vi "App - analyze RUS V6.vi"() -> ()   [LabVIEW 2015] (continued)
"mod time(min)"=58229664.733333334, "file format"=enum."binary", "power(V)"=2.1, "Magn Field(T) "=0.0}, {"temperature"=77.2, "temperature str"="77.20000", "file path"=path "D:/Data/Ultrasound/LSCO/LSCO22__130814c/5_Cooling_2nd_try/September_2014/091714/77.20000K_500_2500_2.10000V_0.00000T_Sep17-2014__02-26-03_001_091714.bin", "last mod"=timestamp(3493779963 s since 1904-01-01), "file name str"="D:\\Data\\Ultrasound\\LSCO\\LSCO22__130814c\\5_Cooling_2nd_try\\September_2014\\091714\\77.20000K_500_2500_2.10000V_0.00000T_Sep17-2014__02-26-03_001_091714.bin", "mod time(min)"=58229666.05, "file format"=enum."binary", "power(V)"=2.1, "Magn Field(T) "=0.0}, {"temperature"=77.118, "temperature str"="77.11800", "file path"=path "D:/Data/Ultrasound/LSCO/LSCO22__130814c/5_Cooling_2nd_try/September_2014/091714/77.11800K_500_2500_2.10000V_0.00000T_Sep17-2014__02-27-22_001_091714.bin", "last mod"=timestamp(3493780042 s since 1904-01-01), "file name str"="D:\\Data\\Ultrasound\\LSCO\\LSCO22__130814c\\5_Cooling_2nd_try\\September_2014\\091714\\77.11800K_500_2500_2.10000V_0.00000T_Sep17-2014__02-27-22_001_091714.bin", "mod time(min)"=58229667.36666667, "file format"=enum."binary", "power(V)"=2.1, "Magn Field(T) "=0.0}, {"temperature"=77.043, "temperature str"="77.04300", "file path"=path "D:/Data/Ultrasound/LSCO/LSCO22__130814c/5_Cooling_2nd_try/September_2014/091714/77.04300K_500_2500_2.10000V_0.00000T_Sep17-2014__02-28-42_001_091714.bin", "last mod"=timestamp(3493780122 s since 1904-01-01), "file name str"="D:\\Data\\Ultrasound\\LSCO\\LSCO22__130814c\\5_Cooling_2nd_try\\September_2014\\091714\\77.04300K_500_2500_2.10000V_0.00000T_Sep17-2014__02-28-42_001_091714.bin", "mod time(min)"=58229668.7, "file format"=enum."binary", "power(V)"=2.1, "Magn Field(T) "=0.0}, {"temperature"=76.965, "temperature str"="76.96500", "file path"=path "D:/Data/Ultrasound/LSCO/LSCO22__130814c/5_Cooling_2nd_try/September_2014/091714/76.96500K_500_2500_2.10000V_0.00000T_Sep17-2014__02-30-01_001_091714.bin", "last mod"=timestamp(3493780201 s since 1904-01-01), "file name str"="D:\\Data\\Ultrasound\\LSCO\\LSCO22__130814c\\5_Cooling_2nd_try\\September_2014\\091714\\76.96500K_500_2500_2.10000V_0.00000T_Sep17-2014__02-30-01_001_091714.bin", "mod time(min)"=58229670.016666666, "file format"=enum."binary", "power(V)"=2.1, "Magn Field(T) "=0.0}, {"temperature"=76.89, "temperature str"="76.89000", "file path"=path "D:/Data/Ultrasound/LSCO/LSCO22__130814c/5_Cooling_2nd_try/September_2014/091714/76.89000K_500_2500_2.10000V_0.00000T_Sep17-2014__02-31-21_001_091714.bin", "last mod"=timestamp(3493780281 s since 1904-01-01), "file name str"="D:\\Data\\Ultrasound\\LSCO\\LSCO22__130814c\\5_Cooling_2nd_try\\September_2014\\091714\\76.89000K_500_2500_2.10000V_0.00000T_Sep17-2014__02-31-21_001_091714.bin", "mod time(min)"=58229671.35, "file format"=enum."binary", "power(V)"=2.1, "Magn Field(T) "=0.0}, {"temperature"=76.811, "temperature str"="76.81100", "file path"=path "D:/Data/Ultrasound/LSCO/LSCO22__130814c/5_Cooling_2nd_try/September_2014/091714/76.81100K_500_2500_2.10000V_0.00000T_Sep17-2014__02-32-40_001_091714.bin", "last mod"=timestamp(3493780360 s since 1904-01-01), "file name str"="D:\\Data\\Ultrasound\\LSCO\\LSCO22__130814c\\5_Cooling_2nd_try\\September_2014\\091714\\76.81100K_500_2500_2.10000V_0.00000T_Sep17-2014__02-32-40_001_091714.bin", "mod time(min)"=58229672.666666664, "file format"=enum."binary", "power(V)"=2.1, "Magn Field(T) "=0.0}, {"temperature"=76.733, "temperature str"="76.73300", "file path"=path "D:/Data/Ultrasound/LSCO/LSCO22__130814c/5_Cooling_2nd_try/September_2014/091714/76.73300K_500_2500_2.10000V_0.00000T_Sep17-2014__02-33-59_001_091714.bin", "last mod"=timestamp(3493780439 s since 1904-01-01), "file name str"="D:\\Data\\Ultrasound\\LSCO\\LSCO22__130814c\\5_Cooling_2nd_try\\September_2014\\091714\\76.73300K_500_2500_2.10000V_0.00000T_Sep17-2014__02-33-59_001_091714.bin", "mod time(min)"=58229673.983333334, "file format"=enum."binary", "power(V)"=2.1, "Magn Field(T) "=0.0}, {"temperature"=76.659, "temperature str"="76.65900", "file path"=path "D:/Data/Ultrasound/LSCO/LSCO22__130814c/5_Cooling_2nd_try/September_2014/091714/76.65900K_500_2500_2.10000V_0.00000T_Sep17-2014__02-35-19_001_091714.bin", "last mod"=timestamp(3493780519 s since 1904-01-01), "file name str"="D:\\Data\\Ultrasound\\LSCO\\LSCO22__130814c\\5_Cooling_2nd_try\\September_2014\\091714\\76.65900K_500_2500_2.10000V_0.00000T_Sep17-2014__02-35-19_001_091714.bin", "mod time(min)"=58229675.31666667, "file format"=enum."binary", "power(V)"=2.1, "Magn Field(T) "=0.0}, {"temperature"=76.581, "temperature str"="76.58100", "file path"=path "D:/Data/Ultrasound/LSCO/LSCO22__130814c/5_Cooling_2nd_try/September_2014/091714/76.58100K_500_2500_2.10000V_0.00000T_Sep17-2014__02-36-38_001_091714.bin", "last mod"=timestamp(3493780598 s since 1904-01-01), "file name str"="D:\\Data\\Ultrasound\\LSCO\\LSCO22__130814c\\5_Cooling_2nd_try\\September_2014\\091714\\76.58100K_500_2500_2.10000V_0.00000T_Sep17-2014__02-36-38_001_091714.bin", "mod time(min)"=58229676.63333333, "file format"=enum."binary", "power(V)"=2.1, "Magn Field(T) "=0.0}, {"temperature"=76.505, "temperature str"="76.50500", "file path"=path "D:/Data/Ultrasound/LSCO/LSCO22__130814c/5_Cooling_2nd_try/September_2014/091714/76.50500K_500_2500_2.10000V_0.00000T_Sep17-2014__02-37-58_001_091714.bin", "last mod"=timestamp(3493780678 s since 1904-01-01), "file name str"="D:\\Data\\Ultrasound\\LSCO\\LSCO22__130814c\\5_Cooling_2nd_try\\September_2014\\091714\\76.50500K_500_2500_2.10000V_0.00000T_Sep17-2014__02-37-58_001_091714.bin", "mod time(min)"=58229677.96666667, "file format"=enum."binary", "power(V)"=2.1, "Magn Field(T) "=0.0}, {"temperature"=76.428, "temperature str"="76.42800", "file path"=path "D:/Data/Ultrasound/LSCO/LSCO22__130814c/5_Cooling_2nd_try/September_2014/091714/76.42800K_500_2500_2.10000V_0.00000T_Sep17-2014__02-39-17_001_091714.bin", "last mod"=timestamp(3493780757 s since 1904-01-01), "file name str"="D:\\Data\\Ultrasound\\LSCO\\LSCO22__130814c\\5_Cooling_2nd_try\\September_2014\\091714\\76.42800K_500_2500_2.10000V_0.00000T_Sep17-2014__02-39-17_001_091714.bin", "mod time(min)"=58229679.28333333, "file format"=enum."binary", "power(V)"=2.1, "Magn Field(T) "=0.0}, {"temperature"=76.351, "temperature str"="76.35100", "file path"=path "D:/Data/Ultrasound/LSCO/LSCO22__130814c/5_Cooling_2nd_try/September_2014/091714/76.35100K_500_2500_2.10000V_0.00000T_Sep17-2014__02-40-36_001_091714.bin", "last mod"=timestamp(3493780836 s since 1904-01-01), "file name str"="D:\\Data\\Ultrasound\\LSCO\\LSCO22__130814c\\5_Cooling_2nd_try\\September_2014\\091714\\76.35100K_500_2500_2.10000V_0.00000T_Sep17-2014__02-40-36_001_091714.bin", "mod time(min)"=58229680.6, "file format"=enum."binary", "power(V)"=2.1, "Magn Field(T) "=0.0}, {"temperature"=76.277, "temperature str"="76.27700", "file path"=path "D:/Data/Ultrasound/LSCO/LSCO22__130814c/5_Cooling_2nd_try/September_2014/091714/76.27700K_500_2500_2.10000V_0.00000T_Sep17-2014__02-41-56_001_091714.bin", "last mod"=timestamp(3493780916 s since 1904-01-01), "file name str"="D:\\Data\\Ultrasound\\LSCO\\LSCO22__130814c\\5_Cooling_2nd_try\\September_2014\\091714\\76.27700K_500_2500_2.10000V_0.00000T_Sep17-2014__02-41-56_001_091714.bin", "mod time(min)"=58229681.93333333, "file format"=enum."binary", "power(V)"=2.1, "Magn Field(T) "=0.0}, {"temperature"=76.2, "temperature str"="76.20000", "file path"=path "D:/Data/Ultrasound/LSCO/LSCO22__130814c/5_Cooling_2nd_try/September_2014/091714/76.20000K_500_2500_2.10000V_0.00000T_Sep17-2014__02-43-15_001_091714.bin", "last mod"=timestamp(3493780995 s since 1904-01-01), "file name str"="D:\\Data\\Ultrasound\\LSCO\\LSCO22__130814c\\5_Cooling_2nd_try\\September_2014\\091714\\76.20000K_500_2500_2.10000V_0.00000T_Sep17-2014__02-43-15_001_091714.bin", "mod time(min)"=58229683.25, "file format"=enum."binary", "power(V)"=2.1, "Magn Field(T) "=0.0}, {"temperature"=76.124, "temperature str"="76.12400", "file path"=path "D:/Data/Ultrasound/LSCO/LSCO22__130814c/5_Cooling_2nd_try/September_2014/091714/76.12400K_500_2500_2.10000V_0.00000T_Sep17-2014__02-44-34_001_091714.bin", "last mod"=timestamp(3493781074 s since 1904-01-01), "file name str"="D:\\Data\\Ultrasound\\LSCO\\LSCO22__130814c\\5_Cooling_2nd_try\\September_2014\\091714\\76.12400K_500_2500_2.10000V_0.00000T_Sep17-2014__02-44-34_001_091714.bin", "mod time(min)"=58229684.56666667, "file format"=enum."binary", "power(V)"=2.1, "Magn Field(T) "=0.0}, {"temperature"=76.051, "temperature str"="76.05100", "file path"=path "D:/Data/Ultrasound/LSCO/LSCO22__130814c/5_Cooling_2nd_try/September_2014/091714/76.05100K_500_2500_2.10000V_0.00000T_Sep17-2014__02-45-54_001_091714.bin", "last mod"=timestamp(3493781154 s since 1904-01-01), "file name str"="D:\\Data\\Ultrasound\\LSCO\\LSCO22__130814c\\5_Cooling_2nd_try\\September_2014\\091714\\76.05100K_500_2500_2.10000V_0.00000T_Sep17-2014__02-45-54_001_091714.bin", "mod time(min)"=58229685.9, "file format"=enum."binary", "power(V)"=2.1, "Magn Field(T) "=0.0}, {"temperature"=75.976, "temperature str"="75.97600", "file path"=path "D:/Data/Ultrasound/LSCO/LSCO22__130814c/5_Cooling_2nd_try/September_2014/091714/75.97600K_500_2500_2.10000V_0.00000T_Sep17-2014__02-47-13_001_091714.bin", "last mod"=timestamp(3493781233 s since 1904-01-01), "file name str"="D:\\Data\\Ultrasound\\LSCO\\LSCO22__130814c\\5_Cooling_2nd_try\\September_2014\\091714\\75.97600K_500_2500_2.10000V_0.00000T_Sep17-2014__02-47-13_001_091714.bin", "mod time(min)"=58229687.21666667, "file format"=enum."binary", "power(V)"=2.1, "Magn Field(T) "=0.0}, {"temperature"=75.901, "temperature str"="75.90100", "file path"=path "D:/Data/Ultrasound/LSCO/LSCO22__130814c/5_Cooling_2nd_try/September_2014/091714/75.90100K_500_2500_2.10000V_0.00000T_Sep17-2014__02-48-33_001_091714.bin", "last mod"=timestamp(3493781313 s since 1904-01-01), "file name str"="D:\\Data\\Ultrasound\\LSCO\\LSCO22__130814c\\5_Cooling_2nd_try\\September_2014\\091714\\75.90100K_500_2500_2.10000V_0.00000T_Sep17-2014__02-48-33_001_091714.bin", "mod time(min)"=58229688.55, "file format"=enum."binary", "power(V)"=2.1, "Magn Field(T) "=0.0}, {"temperature"=75.826, "temperature str"="75.82600", "file path"=path "D:/Data/Ultrasound/LSCO/LSCO22__130814c/5_Cooling_2nd_try/September_2014/091714/75.82600K_500_2500_2.10000V_0.00000T_Sep17-2014__02-49-52_001_091714.bin", "last mod"=timestamp(3493781392 s since 1904-01-01), "file name str"="D:\\Data\\Ultrasound\\LSCO\\LSCO22__130814c\\5_Cooling_2nd_try\\September_2014\\091714\\75.82600K_500_2500_2.10000V_0.00000T_Sep17-2014__02-49-52_001_091714.bin", "mod time(min)"=58229689.86666667, "file format"=enum."binary", "power(V)"=2.1, "Magn Field(T) "=0.0}, {"temperature"=75.75, "temperature str"="75.75000", "file path"=path "D:/Data/Ultrasound/LSCO/LSCO22__130814c/5_Cooling_2nd_try/September_2014/091714/75.75000K_500_2500_2.10000V_0.00000T_Sep17-2014__02-51-11_001_091714.bin", "last mod"=timestamp(3493781471 s since 1904-01-01), "file name str"="D:\\Data\\Ultrasound\\LSCO\\LSCO22__130814c\\5_Cooling_2nd_try\\September_2014\\091714\\75.75000K_500_2500_2.10000V_0.00000T_Sep17-2014__02-51-11_001_091714.bin", "mod time(min)"=58229691.18333333, "file format"=enum."binary", "power(V)"=2.1, "Magn Field(T) "=0.0}, {"temperature"=75.678, "temperature str"="75.67800", "file path"=path "D:/Data/Ultrasound/LSCO/LSCO22__130814c/5_Cooling_2nd_try/September_2014/091714/75.67800K_500_2500_2.10000V_0.00000T_Sep17-2014__02-52-31_001_091714.bin", "last mod"=timestamp(3493781551 s since 1904-01-01), "file name str"="D:\\Data\\Ultrasound\\LSCO\\LSCO22__130814c\\5_Cooling_2nd_try\\September_2014\\091714\\75.67800K_500_2500_2.10000V_0.00000T_Sep17-2014__02-52-31_001_091714.bin", "mod time(min)"=58229692.516666666, "file format"=enum."binary", "power(V)"=2.1, "Magn Field(T) "=0.0}, {"temperature"=75.603, "temperature str"="75.60300", "file path"=path "D:/Data/Ultrasound/LSCO/LSCO22__130814c/5_Cooling_2nd_try/September_2014/091714/75.60300K_500_2500_2.10000V_0.00000T_Sep17-2014__02-53-50_001_091714.bin", "last mod"=timestamp(3493781630 s since 1904-01-01), "file name str"="D:\\Data\\Ultrasound\\LSCO\\LSCO22__130814c\\5_Cooling_2nd_try\\September_2014\\091714\\75.60300K_500_2500_2.10000V_0.00000T_Sep17-2014__02-53-50_001_091714.bin", "mod time(min)"=58229693.833333336, "file format"=enum."binary", "power(V)"=2.1, "Magn Field(T) "=0.0}, {"temperature"=75.531, "temperature str"="75.53100", "file path"=path "D:/Data/Ultrasound/LSCO/LSCO22__130814c/5_Cooling_2nd_try/September_2014/091714/75.53100K_500_2500_2.10000V_0.00000T_Sep17-2014__02-55-09_001_091714.bin", "last mod"=timestamp(3493781709 s since 1904-01-01), "file name str"="D:\\Data\\Ultrasound\\LSCO\\LSCO22__130814c\\5_Cooling_2nd_try\\September_2014\\091714\\75.53100K_500_2500_2.10000V_0.00000T_Sep17-2014__02-55-09_001_091714.bin", "mod time(min)"=58229695.15, "file format"=enum."binary", "power(V)"=2.1, "Magn Field(T) "=0.0}, {"temperature"=75.457, "temperature str"="75.45700", "file path"=path "D:/Data/Ultrasound/LSCO/LSCO22__130814c/5_Cooling_2nd_try/September_2014/091714/75.45700K_500_2500_2.10000V_0.00000T_Sep17-2014__02-56-29_001_091714.bin", "last mod"=timestamp(3493781789 s since 1904-01-01), "file name str"="D:\\Data\\Ultrasound\\LSCO\\LSCO22__130814c\\5_Cooling_2nd_try\\September_2014\\091714\\75.45700K_500_2500_2.10000V_0.00000T_Sep17-2014__02-56-29_001_091714.bin", "mod time(min)"=58229696.483333334, "file format"=enum."binary", "power(V)"=2.1, "Magn Field(T) "=0.0}, {"temperature"=75.379, "temperature str"="75.37900", "file path"=path "D:/Data/Ultrasound/LSCO/LSCO22__130814c/5_Cooling_2nd_try/September_2014/091714/75.37900K_500_2500_2.10000V_0.00000T_Sep17-2014__02-57-48_001_091714.bin", "last mod"=timestamp(3493781868 s since 1904-01-01), "file name str"="D:\\Data\\Ultrasound\\LSCO\\LSCO22__130814c\\5_Cooling_2nd_try\\September_2014\\091714\\75.37900K_500_2500_2.10000V_0.00000T_Sep17-2014__02-57-48_001_091714.bin", "mod time(min)"=58229697.8, "file format"=enum."binary", "power(V)"=2.1, "Magn Field(T) "=0.0}, {"temperature"=75.31, "temperature str"="75.31000", "file path"=path "D:/Data/Ultrasound/LSCO/LSCO22__130814c/5_Cooling_2nd_try/September_2014/091714/75.31000K_500_2500_2.10000V_0.00000T_Sep17-2014__02-59-08_001_091714.bin", "last mod"=timestamp(3493781948 s since 1904-01-01), "file name str"="D:\\Data\\Ultrasound\\LSCO\\LSCO22__130814c\\5_Cooling_2nd_try\\September_2014\\091714\\75.31000K_500_2500_2.10000V_0.00000T_Sep17-2014__02-59-08_001_091714.bin", "mod time(min)"=58229699.13333333, "file format"=enum."binary", "power(V)"=2.1, "Magn Field(T) "=0.0}, {"temperature"=75.236, "temperature str"="75.23600", "file path"=path "D:/Data/Ultrasound/LSCO/LSCO22__130814c/5_Cooling_2nd_try/September_2014/091714/75.23600K_500_2500_2.10000V_0.00000T_Sep17-2014__03-00-27_001_091714.bin", "last mod"=timestamp(3493782027 s since 1904-01-01), "file name str"="D:\\Data\\Ultrasound\\LSCO\\LSCO22__130814c\\5_Cooling_2nd_try\\September_2014\\091714\\75.23600K_500_2500_2.10000V_0.00000T_Sep17-2014__03-00-27_001_091714.bin", "mod time(min)"=58229700.45, "file format"=enum."binary", "power(V)"=2.1, "Magn Field(T) "=0.0}, {"temperature"=75.165, "temperature str"="75.16500", "file path"=path "D:/Data/Ultrasound/LSCO/LSCO22__130814c/5_Cooling_2nd_try/September_2014/091714/75.16500K_500_2500_2.10000V_0.00000T_Sep17-2014__03-01-46_001_091714.bin", "last mod"=timestamp(3493782106 s since 1904-01-01), "file name str"="D:\\Data\\Ultrasound\\LSCO\\LSCO22__130814c\\5_Cooling_2nd_try\\September_2014\\091714\\75.16500K_500_2500_2.10000V_0.00000T_Sep17-2014__03-01-46_001_091714.bin", "mod time(min)"=58229701.766666666, "file format"=enum."binary", "power(V)"=2.1, "Magn Field(T) "=0.0}, {"temperature"=75.09, "temperature str"="75.09000", "file path"=path "D:/Data/Ultrasound/LSCO/LSCO22__130814c/5_Cooling_2nd_try/September_2014/091714/75.09000K_500_2500_2.10000V_0.00000T_Sep17-2014__03-03-06_001_091714.bin", "last mod"=timestamp(3493782186 s since 1904-01-01), "file name str"="D:\\Data\\Ultrasound\\LSCO\\LSCO22__130814c\\5_Cooling_2nd_try\\September_2014\\091714\\75.09000K_500_2500_2.10000V_0.00000T_Sep17-2014__03-03-06_001_091714.bin", "mod time(min)"=58229703.1, "file format"=enum."binary", "power(V)"=2.1, "Magn Field(T) "=0.0}, {"temperature"=75.015, "temperature str"="75.01500", "file path"=path "D:/Data/Ultrasound/LSCO/LSCO22__130814c/5_Cooling_2nd_try/September_2014/091714/75.01500K_500_2500_2.10000V_0.00000T_Sep17-2014__03-04-25_001_091714.bin", "last mod"=timestamp(3493782265 s since 1904-01-01), "file name str"="D:\\Data\\Ultrasound\\LSCO\\LSCO22__130814c\\5_Cooling_2nd_try\\September_2014\\091714\\75.01500K_500_2500_2.10000V_0.00000T_Sep17-2014__03-04-25_001_091714.bin", "mod time(min)"=58229704.416666664, "file format"=enum."binary", "power(V)"=2.1, "Magn Field(T) "=0.0}, {"temperature"=74.945, "temperature str"="74.94500", "file path"=path "D:/Data/Ultrasound/LSCO/LSCO22__130814c/5_Cooling_2nd_try/September_2014/091714/74.94500K_500_2500_2.10000V_0.00000T_Sep17-2014__03-05-45_001_091714.bin", "last mod"=timestamp(3493782345 s since 1904-01-01), "file name str"="D:\\Data\\Ultrasound\\LSCO\\LSCO22__130814c\\5_Cooling_2nd_try\\September_2014\\091714\\74.94500K_500_2500_2.10000V_0.00000T_Sep17-2014__03-05-45_001_091714.bin", "mod time(min)"=58229705.75, "file format"=enum."binary", "power(V)"=2.1, "Magn Field(T) "=0.0}, {"temperature"=74.872, "temperature str"="74.87200", "file path"=path "D:/Data/Ultrasound/LSCO/LSCO22__130814c/5_Cooling_2nd_try/September_2014/091714/74.87200K_500_2500_2.10000V_0.00000T_Sep17-2014__03-07-04_001_091714.bin", "last mod"=timestamp(3493782424 s since 1904-01-01), "file name str"="D:\\Data\\Ultrasound\\LSCO\\LSCO22__130814c\\5_Cooling_2nd_try\\September_2014\\091714\\74.87200K_500_2500_2.10000V_0.00000T_Sep17-2014__03-07-04_001_091714.bin", "mod time(min)"=58229707.06666667, "file format"=enum."binary", "power(V)"=2.1, "Magn Field(T) "=0.0}, {"temperature"=74.801, "temperature str"="74.80100", "file path"=path "D:/Data/Ultrasound/LSCO/LSCO22__130814c/5_Cooling_2nd_try/September_2014/091714/74.80100K_500_2500_2.10000V_0.00000T_Sep17-2014__03-08-23_001_091714.bin", "last mod"=timestamp(3493782503 s since 1904-01-01), "file name str"="D:\\Data\\Ultrasound\\LSCO\\LSCO22__130814c\\5_Cooling_2nd_try\\September_2014\\091714\\74.80100K_500_2500_2.10000V_0.00000T_Sep17-2014__03-08-23_001_091714.bin", "mod time(min)"=58229708.38333333, "file format"=enum."binary", "power(V)"=2.1, "Magn Field(T) "=0.0}, {"temperature"=74.729, "temperature str"="74.72900", "file path"=path "D:/Data/Ultrasound/LSCO/LSCO22__130814c/5_Cooling_2nd_try/September_2014/091714/74.72900K_500_2500_2.10000V_0.00000T_Sep17-2014__03-09-43_001_091714.bin", "last mod"=timestamp(3493782583 s since 1904-01-01), "file name str"="D:\\Data\\Ultrasound\\LSCO\\LSCO22__130814c\\5_Cooling_2nd_try\\September_2014\\091714\\74.72900K_500_2500_2.10000V_0.00000T_Sep17-2014__03-09-43_001_091714.bin", "mod time(min)"=58229709.71666667, "file format"=enum."binary", "power(V)"=2.1, "Magn Field(T) "=0.0}, {"temperature"=74.657, "temperature str"="74.65700", "file path"=path "D:/Data/Ultrasound/LSCO/LSCO22__130814c/5_Cooling_2nd_try/September_2014/091714/74.65700K_500_2500_2.10000V_0.00000T_Sep17-2014__03-11-02_001_091714.bin", "last mod"=timestamp(3493782662 s since 1904-01-01), "file name str"="D:\\Data\\Ultrasound\\LSCO\\LSCO22__130814c\\5_Cooling_2nd_try\\September_2014\\091714\\74.65700K_500_2500_2.10000V_0.00000T_Sep17-2014__03-11-02_001_091714.bin", "mod time(min)"=58229711.03333333, "file format"=enum."binary", "power(V)"=2.1, "Magn Field(T) "=0.0}, {"temperature"=74.584, "temperature str"="74.58400", "file path"=path "D:/Data/Ultrasound/LSCO/LSCO22__130814c/5_Cooling_2nd_try/September_2014/091714/74.58400K_500_2500_2.10000V_0.00000T_Sep17-2014__03-12-21_001_091714.bin", "last mod"=timestamp(3493782741 s since 1904-01-01), "file name str"="D:\\Data\\Ultrasound\\LSCO\\LSCO22__130814c\\5_Cooling_2nd_try\\September_2014\\091714\\74.58400K_500_2500_2.10000V_0.00000T_Sep17-2014__03-12-21_001_091714.bin", "mod time(min)"=58229712.35, "file format"=enum."binary", "power(V)"=2.1, "Magn Field(T) "=0.0}, {"temperature"=74.514, "temperature str"="74.51400", "file path"=path "D:/Data/Ultrasound/LSCO/LSCO22__130814c/5_Cooling_2nd_try/September_2014/091714/74.51400K_500_2500_2.10000V_0.00000T_Sep17-2014__03-13-41_001_091714.bin", "last mod"=timestamp(3493782821 s since 1904-01-01), "file name str"="D:\\Data\\Ultrasound\\LSCO\\LSCO22__130814c\\5_Cooling_2nd_try\\September_2014\\091714\\74.51400K_500_2500_2.10000V_0.00000T_Sep17-2014__03-13-41_001_091714.bin", "mod time(min)"=58229713.68333333, "file format"=enum."binary", "power(V)"=2.1, "Magn Field(T) "=0.0}, {"temperature"=74.444, "temperature str"="74.44400", "file path"=path "D:/Data/Ultrasound/LSCO/LSCO22__130814c/5_Cooling_2nd_try/September_2014/091714/74.44400K_500_2500_2.10000V_0.00000T_Sep17-2014__03-15-00_001_091714.bin", "last mod"=timestamp(3493782900 s since 1904-01-01), "file name str"="D:\\Data\\Ultrasound\\LSCO\\LSCO22__130814c\\5_Cooling_2nd_try\\September_2014\\091714\\74.44400K_500_2500_2.10000V_0.00000T_Sep17-2014__03-15-00_001_091714.bin", "mod time(min)"=58229715.0, "file format"=enum."binary", "power(V)"=2.1, "Magn Field(T) "=0.0}, {"temperature"=74.37, "temperature str"="74.37000", "file path"=path "D:/Data/Ultrasound/LSCO/LSCO22__130814c/5_Cooling_2nd_try/September_2014/091714/74.37000K_500_2500_2.10000V_0.00000T_Sep17-2014__03-16-20_001_091714.bin", "last mod"=timestamp(3493782980 s since 1904-01-01), "file name str"="D:\\Data\\Ultrasound\\LSCO\\LSCO22__130814c\\5_Cooling_2nd_try\\September_2014\\091714\\74.37000K_500_2500_2.10000V_0.00000T_Sep17-2014__03-16-20_001_091714.bin", "mod time(min)"=58229716.333333336, "file format"=enum."binary", "power(V)"=2.1, "Magn Field(T) "=0.0}, {"temperature"=74.299, "temperature str"="74.29900", "file path"=path "D:/Data/Ultrasound/LSCO/LSCO22__130814c/5_Cooling_2nd_try/September_2014/091714/74.29900K_500_2500_2.10000V_0.00000T_Sep17-2014__03-17-39_001_091714.bin", "last mod"=timestamp(3493783059 s since 1904-01-01), "file name str"="D:\\Data\\Ultrasound\\LSCO\\LSCO22__130814c\\5_Cooling_2nd_try\\September_2014\\091714\\74.29900K_500_2500_2.10000V_0.00000T_Sep17-2014__03-17-39_001_091714.bin", "mod time(min)"=58229717.65, "file format"=enum."binary", "power(V)"=2.1, "Magn Field(T) "=0.0}, {"temperature"=74.229, "temperature str"="74.22900", "file path"=path "D:/Data/Ultrasound/LSCO/LSCO22__130814c/5_Cooling_2nd_try/September_2014/091714/74.22900K_500_2500_2.10000V_0.00000T_Sep17-2014__03-18-58_001_091714.bin", "last mod"=timestamp(3493783138 s since 1904-01-01), "file name str"="D:\\Data\\Ultrasound\\LSCO\\LSCO22__130814c\\5_Cooling_2nd_try\\September_2014\\091714\\74.22900K_500_2500_2.10000V_0.00000T_Sep17-2014__03-18-58_001_091714.bin", "mod time(min)"=58229718.96666667, "file format"=enum."binary", "power(V)"=2.1, "Magn Field(T) "=0.0}, {"temperature"=74.159, "temperature str"="74.15900", "file path"=path "D:/Data/Ultrasound/LSCO/LSCO22__130814c/5_Cooling_2nd_try/September_2014/091714/74.15900K_500_2500_2.10000V_0.00000T_Sep17-2014__03-20-18_001_091714.bin", "last mod"=timestamp(3493783218 s since 1904-01-01), "file name str"="D:\\Data\\Ultrasound\\LSCO\\LSCO22__130814c\\5_Cooling_2nd_try\\September_2014\\091714\\74.15900K_500_2500_2.10000V_0.00000T_Sep17-2014__03-20-18_001_091714.bin", "mod time(min)"=58229720.3, "file format"=enum."binary", "power(V)"=2.1, "Magn Field(T) "=0.0}, {"temperature"=74.09, "temperature str"="74.09000", "file path"=path "D:/Data/Ultrasound/LSCO/LSCO22__130814c/5_Cooling_2nd_try/September_2014/091714/74.09000K_500_2500_2.10000V_0.00000T_Sep17-2014__03-21-37_001_091714.bin", "last mod"=timestamp(3493783297 s since 1904-01-01), "file name str"="D:\\Data\\Ultrasound\\LSCO\\LSCO22__130814c\\5_Cooling_2nd_try\\September_2014\\091714\\74.09000K_500_2500_2.10000V_0.00000T_Sep17-2014__03-21-37_001_091714.bin", "mod time(min)"=58229721.61666667, "file format"=enum."binary", "power(V)"=2.1, "Magn Field(T) "=0.0}, {"temperature"=74.017, "temperature str"="74.01700", "file path"=path "D:/Data/Ultrasound/LSCO/LSCO22__130814c/5_Cooling_2nd_try/September_2014/091714/74.01700K_500_2500_2.10000V_0.00000T_Sep17-2014__03-22-56_001_091714.bin", "last mod"=timestamp(3493783376 s since 1904-01-01), "file name str"="D:\\Data\\Ultrasound\\LSCO\\LSCO22__130814c\\5_Cooling_2nd_try\\September_2014\\091714\\74.01700K_500_2500_2.10000V_0.00000T_Sep17-2014__03-22-56_001_091714.bin", "mod time(min)"=58229722.93333333, "file format"=enum."binary", "power(V)"=2.1, "Magn Field(T) "=0.0}, {"temperature"=73.949, "temperature str"="73.94900", "file path"=path "D:/Data/Ultrasound/LSCO/LSCO22__130814c/5_Cooling_2nd_try/September_2014/091714/73.94900K_500_2500_2.10000V_0.00000T_Sep17-2014__03-24-16_001_091714.bin", "last mod"=timestamp(3493783456 s since 1904-01-01), "file name str"="D:\\Data\\Ultrasound\\LSCO\\LSCO22__130814c\\5_Cooling_2nd_try\\September_2014\\091714\\73.94900K_500_2500_2.10000V_0.00000T_Sep17-2014__03-24-16_001_091714.bin", "mod time(min)"=58229724.266666666, "file format"=enum."binary", "power(V)"=2.1, "Magn Field(T) "=0.0}, {"temperature"=73.879, "temperature str"="73.87900", "file path"=path "D:/Data/Ultrasound/LSCO/LSCO22__130814c/5_Cooling_2nd_try/September_2014/091714/73.87900K_500_2500_2.10000V_0.00000T_Sep17-2014__03-25-35_001_091714.bin", "last mod"=timestamp(3493783535 s since 1904-01-01), "file name str"="D:\\Data\\Ultrasound\\LSCO\\LSCO22__130814c\\5_Cooling_2nd_try\\September_2014\\091714\\73.87900K_500_2500_2.10000V_0.00000T_Sep17-2014__03-25-35_001_091714.bin", "mod time(min)"=58229725.583333336, "file format"=enum."binary", "power(V)"=2.1, "Magn Field(T) "=0.0}, {"temperature"=73.808, "temperature str"="73.80800", "file path"=path "D:/Data/Ultrasound/LSCO/LSCO22__130814c/5_Cooling_2nd_try/September_2014/091714/73.80800K_500_2500_2.10000V_0.00000T_Sep17-2014__03-26-55_001_091714.bin", "last mod"=timestamp(3493783615 s since 1904-01-01), "file name str"="D:\\Data\\Ultrasound\\LSCO\\LSCO22__130814c\\5_Cooling_2nd_try\\September_2014\\091714\\73.80800K_500_2500_2.10000V_0.00000T_Sep17-2014__03-26-55_001_091714.bin", "mod time(min)"=58229726.916666664, "file format"=enum."binary", "power(V)"=2.1, "Magn Field(T) "=0.0}, {"temperature"=73.74, "temperature str"="73.74000", "file path"=path "D:/Data/Ultrasound/LSCO/LSCO22__130814c/5_Cooling_2nd_try/September_2014/091714/73.74000K_500_2500_2.10000V_0.00000T_Sep17-2014__03-28-14_001_091714.bin", "last mod"=timestamp(3493783694 s since 1904-01-01), "file name str"="D:\\Data\\Ultrasound\\LSCO\\LSCO22__130814c\\5_Cooling_2nd_try\\September_2014\\091714\\73.74000K_500_2500_2.10000V_0.00000T_Sep17-2014__03-28-14_001_091714.bin", "mod time(min)"=58229728.233333334, "file format"=enum."binary", "power(V)"=2.1, "Magn Field(T) "=0.0}, {"temperature"=73.67, "temperature str"="73.67000", "file path"=path "D:/Data/Ultrasound/LSCO/LSCO22__130814c/5_Cooling_2nd_try/September_2014/091714/73.67000K_500_2500_2.10000V_0.00000T_Sep17-2014__03-29-33_001_091714.bin", "last mod"=timestamp(3493783773 s since 1904-01-01), "file name str"="D:\\Data\\Ultrasound\\LSCO\\LSCO22__130814c\\5_Cooling_2nd_try\\September_2014\\091714\\73.67000K_500_2500_2.10000V_0.00000T_Sep17-2014__03-29-33_001_091714.bin", "mod time(min)"=58229729.55, "file format"=enum."binary", "power(V)"=2.1, "Magn Field(T) "=0.0}, {"temperature"=73.599, "temperature str"="73.59900", "file path"=path "D:/Data/Ultrasound/LSCO/LSCO22__130814c/5_Cooling_2nd_try/September_2014/091714/73.59900K_500_2500_2.10000V_0.00000T_Sep17-2014__03-30-53_001_091714.bin", "last mod"=timestamp(3493783853 s since 1904-01-01), "file name str"="D:\\Data\\Ultrasound\\LSCO\\LSCO22__130814c\\5_Cooling_2nd_try\\September_2014\\091714\\73.59900K_500_2500_2.10000V_0.00000T_Sep17-2014__03-30-53_001_091714.bin", "mod time(min)"=58229730.88333333, "file format"=enum."binary", "power(V)"=2.1, "Magn Field(T) "=0.0}, {"temperature"=73.53, "temperature str"="73.53000", "file path"=path "D:/Data/Ultrasound/LSCO/LSCO22__130814c/5_Cooling_2nd_try/September_2014/091714/73.53000K_500_2500_2.10000V_0.00000T_Sep17-2014__03-32-12_001_091714.bin", "last mod"=timestamp(3493783932 s since 1904-01-01), "file name str"="D:\\Data\\Ultrasound\\LSCO\\LSCO22__130814c\\5_Cooling_2nd_try\\September_2014\\091714\\73.53000K_500_2500_2.10000V_0.00000T_Sep17-2014__03-32-12_001_091714.bin", "mod time(min)"=58229732.2, "file format"=enum."binary", "power(V)"=2.1, "Magn Field(T) "=0.0}, {"temperature"=73.459, "temperature str"="73.45900", "file path"=path "D:/Data/Ultrasound/LSCO/LSCO22__130814c/5_Cooling_2nd_try/September_2014/091714/73.45900K_500_2500_2.10000V_0.00000T_Sep17-2014__03-33-31_001_091714.bin", "last mod"=timestamp(3493784011 s since 1904-01-01), "file name str"="D:\\Data\\Ultrasound\\LSCO\\LSCO22__130814c\\5_Cooling_2nd_try\\September_2014\\091714\\73.45900K_500_2500_2.10000V_0.00000T_Sep17-2014__03-33-31_001_091714.bin", "mod time(min)"=58229733.516666666, "file format"=enum."binary", "power(V)"=2.1, "Magn Field(T) "=0.0}, {"temperature"=73.392, "temperature str"="73.39200", "file path"=path "D:/Data/Ultrasound/LSCO/LSCO22__130814c/5_Cooling_2nd_try/September_2014/091714/73.39200K_500_2500_2.10000V_0.00000T_Sep17-2014__03-34-51_001_091714.bin", "last mod"=timestamp(3493784091 s since 1904-01-01), "file name str"="D:\\Data\\Ultrasound\\LSCO\\LSCO22__130814c\\5_Cooling_2nd_try\\September_2014\\091714\\73.39200K_500_2500_2.10000V_0.00000T_Sep17-2014__03-34-51_001_091714.bin", "mod time(min)"=58229734.85, "file format"=enum."binary", "power(V)"=2.1, "Magn Field(T) "=0.0}, {"temperature"=73.325, "temperature str"="73.32500", "file path"=path "D:/Data/Ultrasound/LSCO/LSCO22__130814c/5_Cooling_2nd_try/September_2014/091714/73.32500K_500_2500_2.10000V_0.00000T_Sep17-2014__03-36-10_001_091714.bin", "last mod"=timestamp(3493784170 s since 1904-01-01), "file name str"="D:\\Data\\Ultrasound\\LSCO\\LSCO22__130814c\\5_Cooling_2nd_try\\September_2014\\091714\\73.32500K_500_2500_2.10000V_0.00000T_Sep17-2014__03-36-10_001_091714.bin", "mod time(min)"=58229736.166666664, "file format"=enum."binary", "power(V)"=2.1, "Magn Field(T) "=0.0}, {"temperature"=73.253, "temperature str"="73.25300", "file path"=path "D:/Data/Ultrasound/LSCO/LSCO22__130814c/5_Cooling_2nd_try/September_2014/091714/73.25300K_500_2500_2.10000V_0.00000T_Sep17-2014__03-37-30_001_091714.bin", "last mod"=timestamp(3493784250 s since 1904-01-01), "file name str"="D:\\Data\\Ultrasound\\LSCO\\LSCO22__130814c\\5_Cooling_2nd_try\\September_2014\\091714\\73.25300K_500_2500_2.10000V_0.00000T_Sep17-2014__03-37-30_001_091714.bin", "mod time(min)"=58229737.5, "file format"=enum."binary", "power(V)"=2.1, "Magn Field(T) "=0.0}, {"temperature"=73.185, "temperature str"="73.18500", "file path"=path "D:/Data/Ultrasound/LSCO/LSCO22__130814c/5_Cooling_2nd_try/September_2014/091714/73.18500K_500_2500_2.10000V_0.00000T_Sep17-2014__03-38-49_001_091714.bin", "last mod"=timestamp(3493784329 s since 1904-01-01), "file name str"="D:\\Data\\Ultrasound\\LSCO\\LSCO22__130814c\\5_Cooling_2nd_try\\September_2014\\091714\\73.18500K_500_2500_2.10000V_0.00000T_Sep17-2014__03-38-49_001_091714.bin", "mod time(min)"=58229738.81666667, "file format"=enum."binary", "power(V)"=2.1, "Magn Field(T) "=0.0}, {"temperature"=73.117, "temperature str"="73.11700", "file path"=path "D:/Data/Ultrasound/LSCO/LSCO22__130814c/5_Cooling_2nd_try/September_2014/091714/73.11700K_500_2500_2.10000V_0.00000T_Sep17-2014__03-40-08_001_091714.bin", "last mod"=timestamp(3493784408 s since 1904-01-01), "file name str"="D:\\Data\\Ultrasound\\LSCO\\LSCO22__130814c\\5_Cooling_2nd_try\\September_2014\\091714\\73.11700K_500_2500_2.10000V_0.00000T_Sep17-2014__03-40-08_001_091714.bin", "mod time(min)"=58229740.13333333, "file format"=enum."binary", "power(V)"=2.1, "Magn Field(T) "=0.0}, {"temperature"=73.048, "temperature str"="73.04800", "file path"=path "D:/Data/Ultrasound/LSCO/LSCO22__130814c/5_Cooling_2nd_try/September_2014/091714/73.04800K_500_2500_2.10000V_0.00000T_Sep17-2014__03-41-28_001_091714.bin", "last mod"=timestamp(3493784488 s since 1904-01-01), "file name str"="D:\\Data\\Ultrasound\\LSCO\\LSCO22__130814c\\5_Cooling_2nd_try\\September_2014\\091714\\73.04800K_500_2500_2.10000V_0.00000T_Sep17-2014__03-41-28_001_091714.bin", "mod time(min)"=58229741.46666667, "file format"=enum."binary", "power(V)"=2.1, "Magn Field(T) "=0.0}, {"temperature"=72.978, "temperature str"="72.97800", "file path"=path "D:/Data/Ultrasound/LSCO/LSCO22__130814c/5_Cooling_2nd_try/September_2014/091714/72.97800K_500_2500_2.10000V_0.00000T_Sep17-2014__03-42-47_001_091714.bin", "last mod"=timestamp(3493784567 s since 1904-01-01), "file name str"="D:\\Data\\Ultrasound\\LSCO\\LSCO22__130814c\\5_Cooling_2nd_try\\September_2014\\091714\\72.97800K_500_2500_2.10000V_0.00000T_Sep17-2014__03-42-47_001_091714.bin", "mod time(min)"=58229742.78333333, "file format"=enum."binary", "power(V)"=2.1, "Magn Field(T) "=0.0}, {"temperature"=72.911, "temperature str"="72.91100", "file path"=path "D:/Data/Ultrasound/LSCO/LSCO22__130814c/5_Cooling_2nd_try/September_2014/091714/72.91100K_500_2500_2.10000V_0.00000T_Sep17-2014__03-44-07_001_091714.bin", "last mod"=timestamp(3493784647 s since 1904-01-01), "file name str"="D:\\Data\\Ultrasound\\LSCO\\LSCO22__130814c\\5_Cooling_2nd_try\\September_2014\\091714\\72.91100K_500_2500_2.10000V_0.00000T_Sep17-2014__03-44-07_001_091714.bin", "mod time(min)"=58229744.11666667, "file format"=enum."binary", "power(V)"=2.1, "Magn Field(T) "=0.0}, {"temperature"=72.846, "temperature str"="72.84600", "file path"=path "D:/Data/Ultrasound/LSCO/LSCO22__130814c/5_Cooling_2nd_try/September_2014/091714/72.84600K_500_2500_2.10000V_0.00000T_Sep17-2014__03-45-26_001_091714.bin", "last mod"=timestamp(3493784726 s since 1904-01-01), "file name str"="D:\\Data\\Ultrasound\\LSCO\\LSCO22__130814c\\5_Cooling_2nd_try\\September_2014\\091714\\72.84600K_500_2500_2.10000V_0.00000T_Sep17-2014__03-45-26_001_091714.bin", "mod time(min)"=58229745.43333333, "file format"=enum."binary", "power(V)"=2.1, "Magn Field(T) "=0.0}, {"temperature"=72.777, "temperature str"="72.77700", "file path"=path "D:/Data/Ultrasound/LSCO/LSCO22__130814c/5_Cooling_2nd_try/September_2014/091714/72.77700K_500_2500_2.10000V_0.00000T_Sep17-2014__03-46-45_001_091714.bin", "last mod"=timestamp(3493784805 s since 1904-01-01), "file name str"="D:\\Data\\Ultrasound\\LSCO\\LSCO22__130814c\\5_Cooling_2nd_try\\September_2014\\091714\\72.77700K_500_2500_2.10000V_0.00000T_Sep17-2014__03-46-45_001_091714.bin", "mod time(min)"=58229746.75, "file format"=enum."binary", "power(V)"=2.1, "Magn Field(T) "=0.0}, {"temperature"=72.707, "temperature str"="72.70700", "file path"=path "D:/Data/Ultrasound/LSCO/LSCO22__130814c/5_Cooling_2nd_try/September_2014/091714/72.70700K_500_2500_2.10000V_0.00000T_Sep17-2014__03-48-05_001_091714.bin", "last mod"=timestamp(3493784885 s since 1904-01-01), "file name str"="D:\\Data\\Ultrasound\\LSCO\\LSCO22__130814c\\5_Cooling_2nd_try\\September_2014\\091714\\72.70700K_500_2500_2.10000V_0.00000T_Sep17-2014__03-48-05_001_091714.bin", "mod time(min)"=58229748.083333336, "file format"=enum."binary", "power(V)"=2.1, "Magn Field(T) "=0.0}, {"temperature"=72.643, "temperature str"="72.64300", "file path"=path "D:/Data/Ultrasound/LSCO/LSCO22__130814c/5_Cooling_2nd_try/September_2014/091714/72.64300K_500_2500_2.10000V_0.00000T_Sep17-2014__03-49-24_001_091714.bin", "last mod"=timestamp(3493784964 s since 1904-01-01), "file name str"="D:\\Data\\Ultrasound\\LSCO\\LSCO22__130814c\\5_Cooling_2nd_try\\September_2014\\091714\\72.64300K_500_2500_2.10000V_0.00000T_Sep17-2014__03-49-24_001_091714.bin", "mod time(min)"=58229749.4, "file format"=enum."binary", "power(V)"=2.1, "Magn Field(T) "=0.0}, {"temperature"=72.574, "temperature str"="72.57400", "file path"=path "D:/Data/Ultrasound/LSCO/LSCO22__130814c/5_Cooling_2nd_try/September_2014/091714/72.57400K_500_2500_2.10000V_0.00000T_Sep17-2014__03-50-43_001_091714.bin", "last mod"=timestamp(3493785043 s since 1904-01-01), "file name str"="D:\\Data\\Ultrasound\\LSCO\\LSCO22__130814c\\5_Cooling_2nd_try\\September_2014\\091714\\72.57400K_500_2500_2.10000V_0.00000T_Sep17-2014__03-50-43_001_091714.bin", "mod time(min)"=58229750.71666667, "file format"=enum."binary", "power(V)"=2.1, "Magn Field(T) "=0.0}, {"temperature"=72.507, "temperature str"="72.50700", "file path"=path "D:/Data/Ultrasound/LSCO/LSCO22__130814c/5_Cooling_2nd_try/September_2014/091714/72.50700K_500_2500_2.10000V_0.00000T_Sep17-2014__03-52-03_001_091714.bin", "last mod"=timestamp(3493785123 s since 1904-01-01), "file name str"="D:\\Data\\Ultrasound\\LSCO\\LSCO22__130814c\\5_Cooling_2nd_try\\September_2014\\091714\\72.50700K_500_2500_2.10000V_0.00000T_Sep17-2014__03-52-03_001_091714.bin", "mod time(min)"=58229752.05, "file format"=enum."binary", "power(V)"=2.1, "Magn Field(T) "=0.0}, {"temperature"=72.439, "temperature str"="72.43900", "file path"=path "D:/Data/Ultrasound/LSCO/LSCO22__130814c/5_Cooling_2nd_try/September_2014/091714/72.43900K_500_2500_2.10000V_0.00000T_Sep17-2014__03-53-22_001_091714.bin", "last mod"=timestamp(3493785202 s since 1904-01-01), "file name str"="D:\\Data\\Ultrasound\\LSCO\\LSCO22__130814c\\5_Cooling_2nd_try\\September_2014\\091714\\72.43900K_500_2500_2.10000V_0.00000T_Sep17-2014__03-53-22_001_091714.bin", "mod time(min)"=58229753.36666667, "file format"=enum."binary", "power(V)"=2.1, "Magn Field(T) "=0.0}, {"temperature"=72.371, "temperature str"="72.37100", "file path"=path "D:/Data/Ultrasound/LSCO/LSCO22__130814c/5_Cooling_2nd_try/September_2014/091714/72.37100K_500_2500_2.10000V_0.00000T_Sep17-2014__03-54-42_001_091714.bin", "last mod"=timestamp(3493785282 s since 1904-01-01), "file name str"="D:\\Data\\Ultrasound\\LSCO\\LSCO22__130814c\\5_Cooling_2nd_try\\September_2014\\091714\\72.37100K_500_2500_2.10000V_0.00000T_Sep17-2014__03-54-42_001_091714.bin", "mod time(min)"=58229754.7, "file format"=enum."binary", "power(V)"=2.1, "Magn Field(T) "=0.0}, {"temperature"=72.308, "temperature str"="72.30800", "file path"=path "D:/Data/Ultrasound/LSCO/LSCO22__130814c/5_Cooling_2nd_try/September_2014/091714/72.30800K_500_2500_2.10000V_0.00000T_Sep17-2014__03-56-01_001_091714.bin", "last mod"=timestamp(3493785361 s since 1904-01-01), "file name str"="D:\\Data\\Ultrasound\\LSCO\\LSCO22__130814c\\5_Cooling_2nd_try\\September_2014\\091714\\72.30800K_500_2500_2.10000V_0.00000T_Sep17-2014__03-56-01_001_091714.bin", "mod time(min)"=58229756.016666666, "file format"=enum."binary", "power(V)"=2.1, "Magn Field(T) "=0.0}, {"temperature"=72.238, "temperature str"="72.23800", "file path"=path "D:/Data/Ultrasound/LSCO/LSCO22__130814c/5_Cooling_2nd_try/September_2014/091714/72.23800K_500_2500_2.10000V_0.00000T_Sep17-2014__03-57-20_001_091714.bin", "last mod"=timestamp(3493785440 s since 1904-01-01), "file name str"="D:\\Data\\Ultrasound\\LSCO\\LSCO22__130814c\\5_Cooling_2nd_try\\September_2014\\091714\\72.23800K_500_2500_2.10000V_0.00000T_Sep17-2014__03-57-20_001_091714.bin", "mod time(min)"=58229757.333333336, "file format"=enum."binary", "power(V)"=2.1, "Magn Field(T) "=0.0}, {"temperature"=72.173, "temperature str"="72.17300", "file path"=path "D:/Data/Ultrasound/LSCO/LSCO22__130814c/5_Cooling_2nd_try/September_2014/091714/72.17300K_500_2500_2.10000V_0.00000T_Sep17-2014__03-58-40_001_091714.bin", "last mod"=timestamp(3493785520 s since 1904-01-01), "file name str"="D:\\Data\\Ultrasound\\LSCO\\LSCO22__130814c\\5_Cooling_2nd_try\\September_2014\\091714\\72.17300K_500_2500_2.10000V_0.00000T_Sep17-2014__03-58-40_001_091714.bin", "mod time(min)"=58229758.666666664, "file format"=enum."binary", "power(V)"=2.1, "Magn Field(T) "=0.0}, {"temperature"=72.106, "temperature str"="72.10600", "file path"=path "D:/Data/Ultrasound/LSCO/LSCO22__130814c/5_Cooling_2nd_try/September_2014/091714/72.10600K_500_2500_2.10000V_0.00000T_Sep17-2014__03-59-59_001_091714.bin", 
